vi "PAC-SLI.vi"() -> ()   [LabVIEW 2017]
uses:
  <vilib>/MakerHub/LINX/Private/Type Defs/Peripherals/SPI/SPI Configuration.ctl
  <vilib>/MakerHub/LINX/Private/Type Defs/Peripherals/SPI/SPI Bit Order.ctl
  <vilib>/MakerHub/LINX/Private/Type Defs/Peripherals/SPI/SPI Mode.ctl
  <vilib>/MakerHub/LINX/Public/Peripherals/SPI/SPI CS Config.ctl
  <vilib>/MakerHub/LINX/Private/Type Defs/Peripherals/SPI/SPI CS Logic Level.ctl
  <vilib>/Analysis/Matrix/Datatypes/RealMatrix.ctl
  <vilib>/MakerHub/LINX/Public/Peripherals/PWM/PWM Set Duty Cycle 1 Chan.vi
  <vilib>/MakerHub/LINX/Public/Peripherals/Analog/Analog Read 1 Chan.vi
  <vilib>/MakerHub/LINX/Public/Peripherals/Analog/Analog Read N Chans.vi
  <vilib>/MakerHub/LINX/Private/Local IO/LinxAnalogRead.vi
  <vilib>/MakerHub/LINX/Public/Utilities/Check Channel.vi
  <vilib>/MakerHub/LINX/Public/Utilities/Open Serial.vi
  <vilib>/MakerHub/LINX/Public/Peripherals/PWM/PWM Set Duty Cycle N Chans.vi
  <vilib>/MakerHub/LINX/Private/Utilties/Generate Error.vi
  <vilib>/Analysis/Matrix/Numeric/Conversions/Matrix To Array - RM.vi
  <vilib>/MakerHub/LINX/LMH-LINX.lvlib
  <vilib>/Analysis/Matrix/NI_Matrix.lvlib
panel:
  in  "START Button":bool
  out "stop 2":bool
  out "Connection Initialized":bool
  out "Debug console":string
  in  "reset":bool
  in  "stop":bool
  out "I/O Device Name":string
  in  "?":T1(tab)
  in  "StayON 6":bool
  in  "StayON 5":bool
  in  "StayON 4":bool
  in  "StayON 3":bool
  in  "StayON 2":bool
  in  "StayON 1":bool
  in  "Detector  6":bool
  out "Det 6 status":bool
  in  "Detector  5":bool
  out "Det 5 status":bool
  in  "Detector  4":bool
  out "Det 4 status":bool
  in  "Detector 3":bool
  out "Det 3 status":bool
  in  "Detector 2":bool
  out "Det 2 status":bool
  in  "Detector 1":bool
  out "Det 1 status":bool
  out "Photogate AIN":u8
  out "Stepper PUL DOUT":u8
  out "Stepper DIR DOUT":u8
  out "Stepper ENA DOUT":u8
  out "DigiPAC UART":u8
  out "Thermocouple 1":string
  out "Thermocouple 2":string
  out "Furnace ctrl Channel":u8
  out "Beam gate channel":u8
  in  "Furnace power% set":u8 max=100
  out "Furnace power%":u8
  out "Elapsed Super\nCycle Time (s)":dbl caption="Elapsed Time (s)"
  in  "Supercycle time [s]":dbl
  in  "CS Configuration":T2={"CS Channel"=7, "CS Logic Level"=enum."Active High"}
  in  "SPI Configuration":T4={"Clock Frequency"=1000000, "Bit Order"=enum."LSb First", "SPI Mode"=enum."Mode 0"}
  out "Clock Frequency":u32
  in  "CS Configuration 2":T2={"CS Channel"=7, "CS Logic Level"=enum."Active High"}
  in  "Photogate AIN":u8
  in  "Stepper PUL DOUT":u8
  in  "Stepper DIR DOUT":u8
  in  "Stepper ENA DOUT":u8
  in  "DigiPAC UART":u8
  in  "Furnace ctrl Channel":u8=9 min=9 max=10
  in  "Beam gate channel":u8
  in  "Operation|Time":T7
  in  "Serial Port":refnum<visa-resource-name>="COM3"
  # "Check settings before running!"
  # "I/O Channels"
  # "Temperature"
  # "Set      Status"
  # "Furnace power output"
  # "DIN.............."
  # "Digital input"
  # "DOUT.........."
  # "Digital output"
  # "AIN.............."
  # "Analog input"
  # "UART..........."
  # "Serial port"
  # "I/O ports"
  # "Thermocouple SPI settings"
  # "Automation order and timing"
  # "Thermocouple SPI settings required by MAX31855 amplifier:\nCS Logic level.............Active Low\nBit Order......................MSb First\nSPI Mode.....................Mode 0\nClock Frequency........<15000000\n                                      12500 is ok\nMISO/Data port...........50\nCLK port.......................52"
  # "Operation command numbers\n0, No action\n1, Detector acq. ON\n2, Detector acq. OFF\n3, Furnace power set\n4, Beam gate OFF\n5, Beam gate ON\n6, Furnace position IN\n7, Furnace position OUT\n8, Detector status check"
  # "Furnace control\nChannel forced\nto 9 or 10 due\nhardware setup\nin firmware.\nMore information in \ndocumentation"
  # "Author: Mikko Kivekäs\nVersion: 0.2.0\nDate: 07/2019\nLicense: GPLv3\n\nThis program is created for PAC-SLI measurement setup in ISOLDE, CERN. This program is created for research use and should not be used in commercial applications.\n\nThis program is designed to be operated with Arduino Mega2560 I/O-board.  Communication between Arduino and this LabVIEW program uses serial communication over USB. MakerHub LINX library is used. https://www.labviewmakerhub.com/doku.php?id=libraries:linx:start\n\n\nIn monitoring tab user can monitor input and output values. Monitoring tab has also the control of detector data acquisition control. \n\nSettings tab contains all essential settings for running the measurement automation. There user can control I/O-ports, SPI settings and automation operation order and timing. SPI is used to read temperature values from MAX31855KASA+ thermocouple amplifier-adc. SPI MISO and CLK ports are fixed due Arduino design and stated under SPI-settings.\n\n     I/O type.....................I/O-port\n     -MISO/DO/Data.......50\n     -CLK/Clock...............52\n\nFurnace power setting I/O-port must be digital I/O-port with PMW. Choose of digital ports 2-13 (Arduino Mega2560). \n\nIndicator next to device name is ON when link between PC and Arduino is established and ready to run. Spress Start-button to run.\n\nCAUTION! FURNACE MUST BE IN UP POSITION, OTHERWISE FURNACE WILL BREAK DURING RUN.\n\nIf program does not run normally or you press \"Abort Execution\" of LabVIEW, build firmware to Arduino again. It is good practice to build firmware before\nevery run start. One can build firmware in LabVIEW going \n\n    Tools >> MakerHUB >> LINX >> LINX Firmware Wizard...  \n\nand there choosing right I/O-board and communication channel. In case of firmware not installing properly, disconnect all wires from Arduino, go to Arduino \nIDE and build in empty Sketch. If that does uploads properly, you can proceed to build LINX firmware.\n\nYou can find VIs and other information from https://github.com/MikkoKivekas/PAC-SLI\n\nThis program uses custom LINX firmware, read more from README."
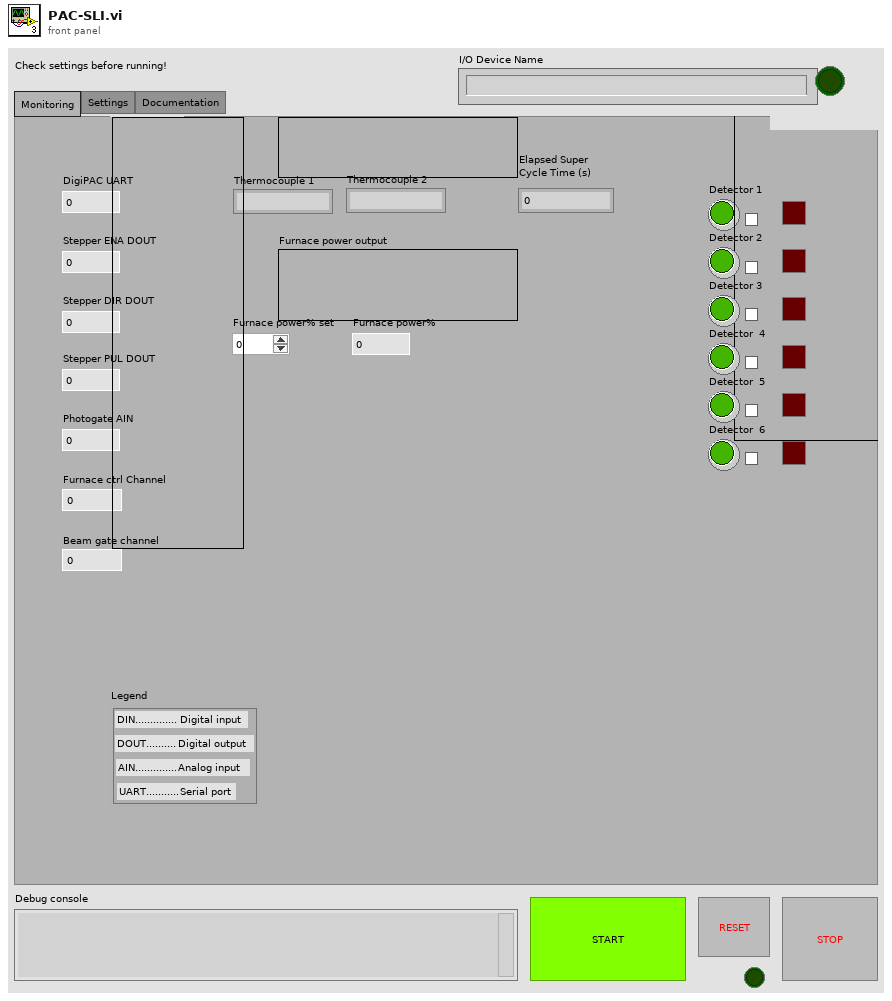
[diagram p1: front panel]
types:
  T1 = enum32{"Monitoring", "Settings", "Documentation"}
  T2 = typedef "LMH-LINX.lvlib/SPI CS Config.ctl" = cluster{"CS Channel":u8, "CS Logic Level":T3}
  T3 = typedef "LMH-LINX.lvlib/SPI CS Logic Level.ctl" = enum8{"Active Low", "Active High"}
  T4 = typedef "LMH-LINX.lvlib/SPI Configuration.ctl" = cluster{"Clock Frequency":u32, "Bit Order":T5, "SPI Mode":T6}
  T5 = typedef "LMH-LINX.lvlib/SPI Bit Order.ctl" = enum8{"LSb First", "MSb First"}
  T6 = typedef "LMH-LINX.lvlib/SPI Mode.ctl" = enum8{"Mode 0", "Mode 1", "Mode 2", "Mode 3"}
  T7 = typedef "NI_Matrix.lvlib/RealMatrix.ctl" = dbl[][]
  T8 = typedef "LMH-LINX.lvlib/LINX Ref.ctl" = cluster{"IO":T9, "Interface":T10, "LINX Device Config":T11}
  T9 = typedef "LMH-LINX.lvlib/Platform.ctl" = enum16{"Remote", "Local"}
  T10 = typedef "LMH-LINX.lvlib/Interface.ctl" = enum16{"Serial", "TCP"}
  T11 = typedef "LMH-LINX.lvlib/Device.lvlib/LINX Device Config.ctl" = cluster{"Interface":T10, "COM Port":refnum<visa-resource-name>, "TCP Configuration":T12, "Device Family":u8, "Device ID":u8, "Device Name":string, "TCP Ref":refnum<k5>, "Channels":T13}
  T12 = typedef "LMH-LINX.lvlib/Device.lvlib/TCP Config.ctl" = cluster{"IP Address":string, "Port":u16}
  T13 = typedef "LMH-LINX.lvlib/Channels.ctl" = cluster{"DI":u8[], "DO":u8[], "AI":u8[], "AO":u8[], "PWM":u8[], "QE":u8[], "UART":u8[], "I2C 2":u8[], "SPI":u8[], "CAN":u8[], "Servo":u8[], "AI Ref (V)":dbl, "AI Resolution (Bits)":u8, "AO Ref (V)":dbl, "AO Resolution (Bits)":u8}
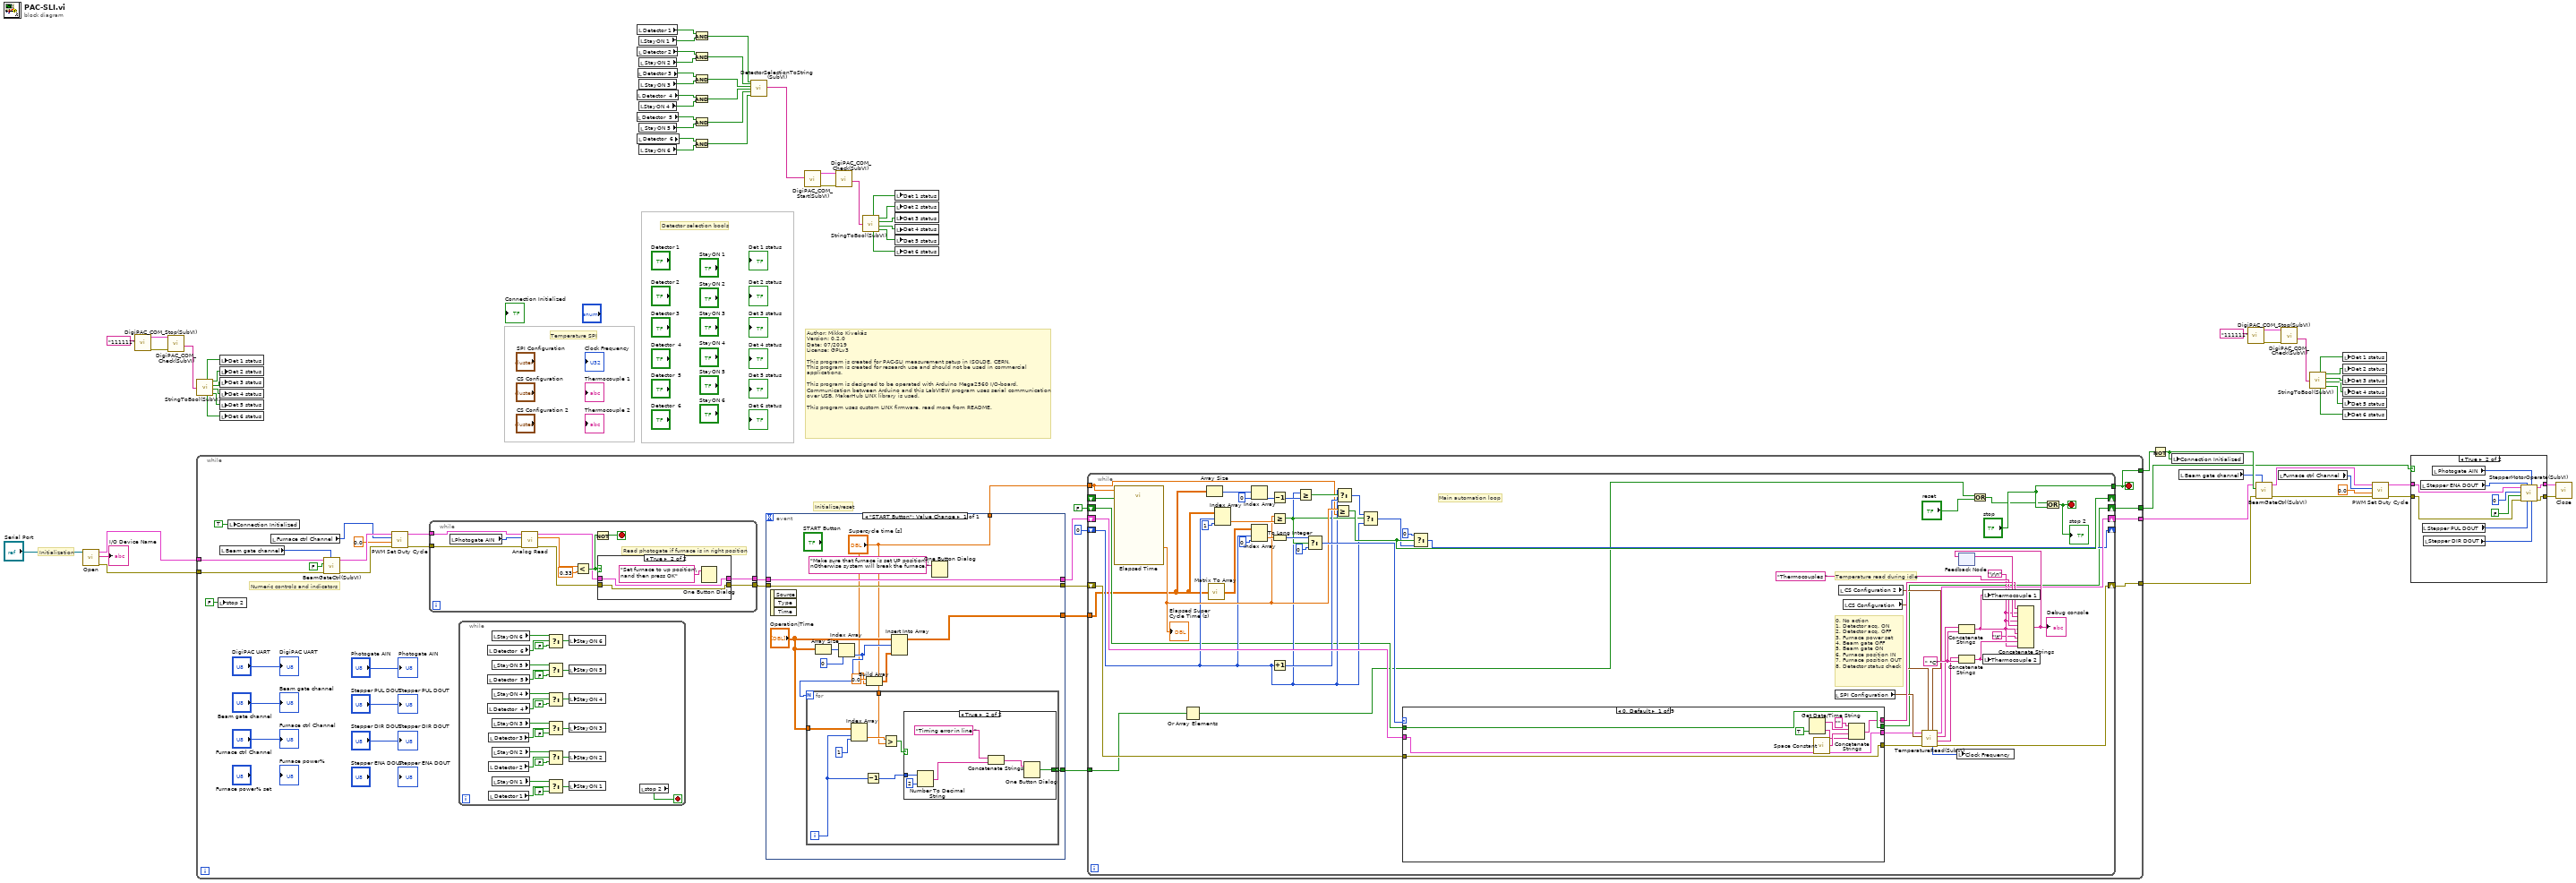
[diagram p0: block diagram]
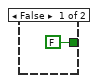
[diagram p4: hidden frame]
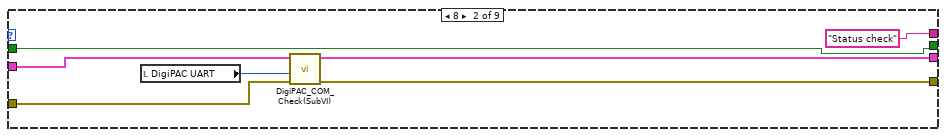
[diagram p5: hidden frame]
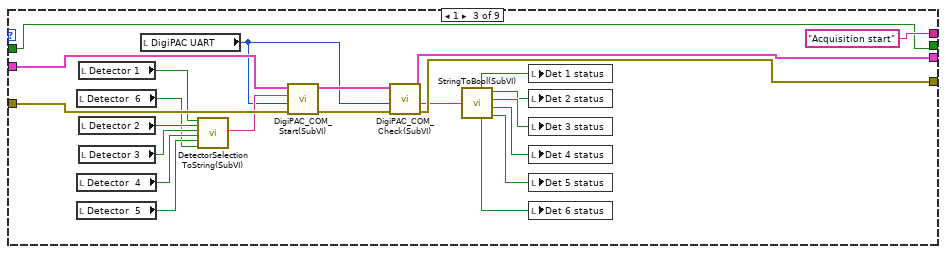
[diagram p6: hidden frame]
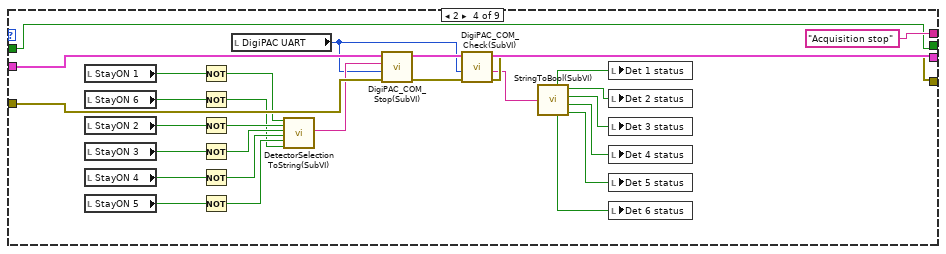
[diagram p7: hidden frame]
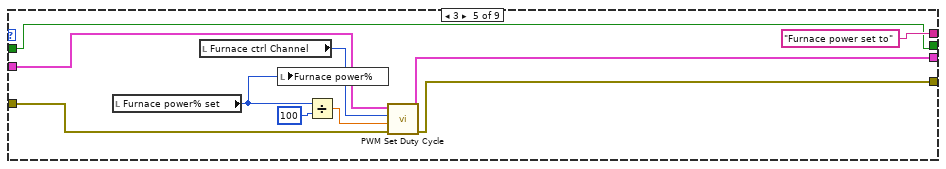
[diagram p8: hidden frame]
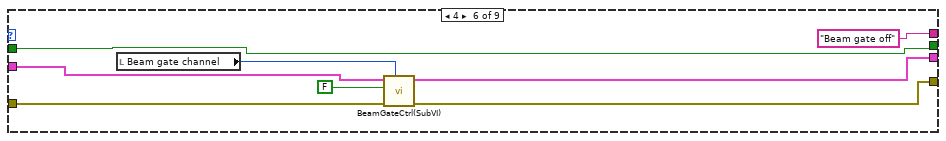
[diagram p9: hidden frame]
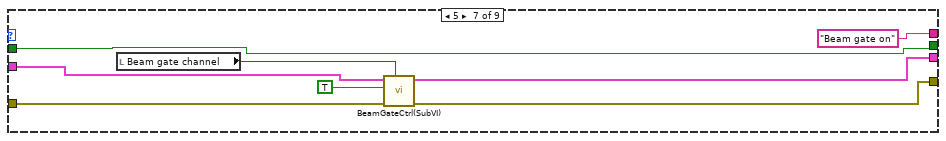
[diagram p10: hidden frame]
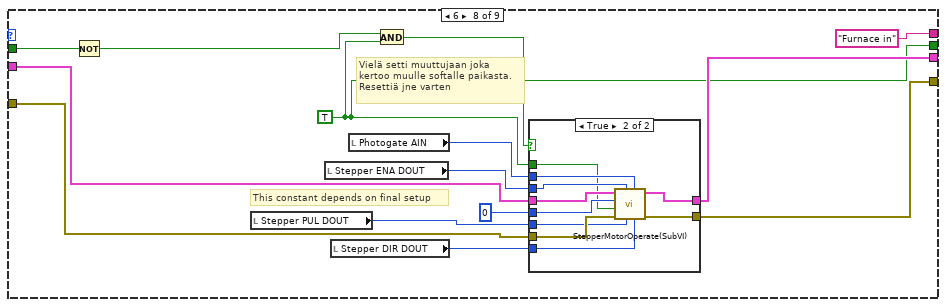
[diagram p11: hidden frame]
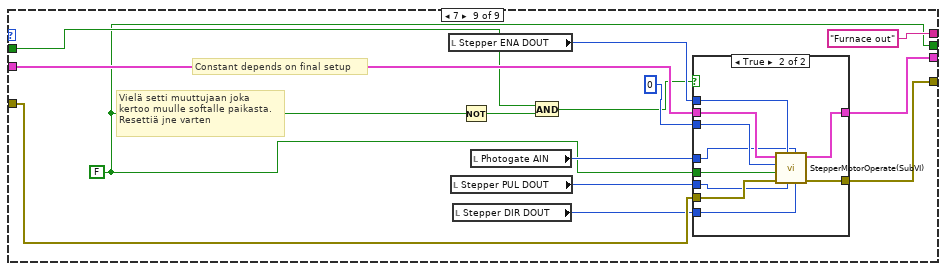
[diagram p13: hidden frame]
diagram:
  # "Author: Mikko Kivekäs\nVersion: 0.2.0\nDate: 07/2019\nLicense: GPLv3\n\nThis program is created for PAC-SLI measurement setup in ISOLDE, CERN.\nThis program is created for research use and should not be used in commercial\napplications.\n\nThis program is designed to be operated with Arduino Mega2560 I/O-board. \nCommunication between Arduino and this LabVIEW program uses serial communication\nover USB. MakerHub LINX library is used.\n\nThis program uses custom LINX firmware, read more from README."
  # "Initialization"
  # "Temperature SPI"
  # "Detector selection bools"
  n1 = call-poly <vilib>:"Open.vi"("Serial Port"="Serial Port") -> ("Error Out"=w63:errorcluster, "Device Name"=→"I/O Device Name":string, "LINX Resource"=w64:T8)  [unwired: 8 in]
  n2 = call "DigiPAC_COM_Stop(SubVI).vi"("Detector input"="111111") -> ("error out"=w37:errorcluster, "LINX Resource out"=w38:T8)  [unwired: 8 in, 1 out]
  n3 = call "DigiPAC_COM_Check(SubVI).vi"("error in (no error)"=w37, "LINX Resource in"=w38) -> ("Confirmation message"=w35:string)  [unwired: 6 in, 3 out]
  n4 = call "StringToBool(SubVI).vi"("string"=w35) -> ("Det 1"=w27:bool, "Det 2"=w26:bool, "Det 3"=w25:bool, "Det 6"=w22:bool, "Det 4"=w24:bool, "Det 5"=w23:bool)  [unwired: 4 in]
  n5 = while {
    tunnel: w64 -> [w83]
    tunnel: w63 -> [w82]
    tunnel: [w96] -> w59
    tunnel: [w95] -> w58
    tunnel: [w77] -> w62
    tunnel: [w91] -> w49
    stop <- w77 stop-if-true
    # "Numeric controls and indicators"
    # "Initialize/reset"
    n6 = local write "stop 2"(FALSE ("stop 2")) -> ()
    n7 = local read "Beam gate channel"() -> (w78:u8)
    n8 = local write "Connection Initialized"(TRUE ("Connection Initialized")) -> ()
    n9 = local read "Furnace ctrl Channel"() -> (w79:u8)
    n10 = call "BeamGateCtrl(SubVI).vi"("Beam gate ctrl channel"=w78, "Error In"=w82, "Output Value"=FALSE, "LINX Resource"=w83) -> ("Error Out"=w86:errorcluster, "LINX Resource 2"=w87:T8)  [unwired: 6 in]
    n11 = call-poly <vilib>:"PWM Set Duty Cycle.vi"("Error In"=w86, "Duty Cycle (0-1)"=0.0, "PWM Channel"=w79, "LINX Resource"=w87) -> ("Error Out"=w84:errorcluster, "LINX Resource"=w85:T8)  [unwired: 6 in]
    n12 = while {
      tunnel: w85 -> [w128]
      tunnel: [w126] -> w89
      tunnel: w84 -> [w125]
      tunnel: [w123] -> w88
      stop <- w129 stop-if-true
      # "Read photogate if furnace is in right position"
      n13 = local read "Photogate AIN"() -> (w131:u8)
      n14 = call-poly <vilib>:"Analog Read.vi"("Error In"=w125, "Analog Channel"=w131, "LINX Resource"=w128) -> ("Error Out"=w124:errorcluster, "Voltage"=w133:dbl, "LINX Resource"=w127:T8)  [unwired: 5 in, 1 out]
      n15 = Less?(x=w133, y=0.33) -> (x < y?=w130:bool)
      n16 = Not(x=w130) -> (.not. x?=w129:bool)
      n17 = case shown="True" w130 {
        tunnel: w127 -> [w135 w137]
        tunnel: [w135 w137] -> w126
        tunnel: w124 -> [w134 w136]
        tunnel: [w134 w136] -> w123
        frame False {
        }
        frame True {
          n18 = One Button Dialog(message="Set furnace to up position\nand then press OK") -> ()  [unwired: 1 in, 1 out]
        }
      }
    }
    n19 = while {
      stop <- w98 stop-if-true
      n20 = local read "Detector  6"() -> (w121:bool)
      n21 = local read "Detector  5"() -> (w119:bool)
      n22 = local read "Detector  4"() -> (w117:bool)
      n23 = local read "Detector 3"() -> (w115:bool)
      n24 = local read "Detector 2"() -> (w113:bool)
      n25 = local read "Detector 1"() -> (w111:bool)
      n26 = local read "StayON 6"() -> (w122:bool)
      n27 = local read "StayON 5"() -> (w120:bool)
      n28 = local read "StayON 4"() -> (w118:bool)
      n29 = local read "StayON 3"() -> (w116:bool)
      n30 = local read "StayON 2"() -> (w114:bool)
      n31 = local read "StayON 1"() -> (w112:bool)
      n32 = Select(t=w122, s=w121, f=FALSE) -> (s? t:f=w110:bool)
      n33 = Select(t=w120, s=w119, f=FALSE) -> (s? t:f=w109:bool)
      n34 = Select(t=w118, s=w117, f=FALSE) -> (s? t:f=w108:bool)
      n35 = Select(t=w116, s=w115, f=FALSE) -> (s? t:f=w107:bool)
      n36 = Select(t=w114, s=w113, f=FALSE) -> (s? t:f=w106:bool)
      n37 = Select(t=w112, s=w111, f=FALSE) -> (s? t:f=w105:bool)
      n38 = local write "StayON 6"(w110) -> ()
      n39 = local write "StayON 5"(w109) -> ()
      n40 = local write "StayON 4"(w108) -> ()
      n41 = local write "StayON 3"(w107) -> ()
      n42 = local write "StayON 2"(w106) -> ()
      n43 = local write "StayON 1"(w105) -> ()
      n44 = local read "stop 2"() -> (w98:bool)
    }
    n45 = event shown="[0] \"START Button\": Value Change" {
      selector: _ -> [_]
      dyn-events: _ -> [_]
      timeout: _ -> [_]
      tunnel: w89 -> [w149]
      tunnel: [w149] -> w94
      tunnel: w88 -> [w148]
      tunnel: [w148] -> w93
      tunnel: ["Supercycle time [s]"] -> w70
      tunnel: [w145] -> w68
      tunnel: [w139] -> w67
      event "START Button": Value Change {
        n46 = event-data() -> ()  [unwired: 1 in, 3 out]
        n47 = Array Size(array="Operation|Time") -> (size(s)=w144:i32[])
        n48 = Index Array(array=w144, index=0) -> (element=w142:i32)
        n49 = for {
          N: w142 -> [_]
          tunnel: "Operation|Time" -> [w158]
          tunnel: "Supercycle time [s]" -> [w155]
          tunnel: [w153] -> w139 mode=indexing
          i -> [w152]
          n50 = Index Array(array=w158, index (row)=w152, index (col)=1 ("disabled index (col)")) -> (element=w156:dbl)
          n51 = Decrement(x=w152) -> (x-1=w151:i32)
          n52 = Greater?(x=w156, y=w155) -> (0:w154:bool)
          n53 = case shown="True" w154 {
            tunnel: w151 -> [_ w165]
            tunnel: [FALSE ("true") w160] -> w153
            frame False {
            }
            frame True {
              n54 = Number To Decimal String(number=w165, width (-)=i16 2) -> (decimal integer string=w164:string)
              n55 = Concatenate Strings("Timing error in line ", w164) -> (w161:string)
              n56 = One Button Dialog(message=w161) -> (true=w160:bool)  [unwired: 1 in]
            }
          }
        }
        n57 = Build Array(0.0, "Supercycle time [s]") -> (w147:T7)
        n58 = Insert Into Array(array="Operation|Time", index (row)=w142, new element=w147) -> (w145:T7)  [unwired: 1 in]
        n59 = One Button Dialog(message="Make sure that furnace is set UP position.\nOtherwise system will break the furnace.") -> ()  [unwired: 1 in, 1 out]
      }
    }
    n60 = while {
      tunnel: ["stop"] -> w77
      shift-right: [w177] -> _
      shift-left: 0 -> [w176]
      shift-right: [w202] -> w96
      shift-left: w94 -> [w219]
      shift-right: [w201] -> w95
      shift-left: w93 -> [w218]
      shift-right: [w184] -> _
      shift-left: _ -> [w185]
      shift-right: [w175] -> w91
      shift-left: FALSE ("Direction input") -> [w174]
      tunnel: w70 -> [w173]
      tunnel: w68 -> [w171]
      tunnel: w67 -> [w170]
      stop <- w172 stop-if-true
      w188 = "\r\n"
      w213 = " °C"
      # "0, No action\n1, Detector acq. ON\n2, Detector acq. OFF\n3, Furnace power set\n4, Beam gate OFF\n5, Beam gate ON\n6, Furnace position IN\n7, Furnace position OUT\n8, Detector status check"
      # "Temperature read during idle"
      # "Main automation loop"
      n61 = call "Elapsed Time"("Time Target (s)"=w173, "Reset"=w185) -> ("Elapsed Time (s)"=w186:dbl)  [unwired: 10 in, 7 out]
      "Elapsed Super\nCycle Time (s)" <- w186
      n62 = Or Array Elements(Boolean array=w170) -> (logical OR=w168:bool)
      n63 = Array Size(array=w171) -> (size(s)=w217:i32[])
      n64 = call-poly <vilib>:"Matrix To Array.vi"("Real Matrix"=w171) -> ("Real 2D Array"=w215:dbl[][])
      n65 = Index Array(array=w171, index (row)=w176, index (col)=1 ("disabled index (col)")) -> (element=w195:dbl)
      n66 = Index Array(array=w217, index=0) -> (element=w210:i32)
      n67 = Index Array(array=w215, index (row)=w176, index (col)=0 ("disabled index (col)")) -> (element=w212:dbl)
      n68 = Decrement(x=w210) -> (x-1=w211:i32)
      n69 = Greater Or Equal?(x=w186, y=w195) -> (x >= y?=w179:bool)
      n70 = To Long Integer(number=w212) -> (32bit integer=w194:i32)
      n71 = Increment(x=w176) -> (x+1=w182:i32)
      n72 = Greater Or Equal?(x=w176, y=w211) -> (x >= y?=w181:bool)
      n73 = Select(t=w194, s=w179, f=0) -> (s? t:f=w192:i32)
      n74 = Greater Or Equal?(x=w186, y=w173) -> (x >= y?=w184:bool)
      n75 = Select(t=w176, s=w181, f=w182) -> (s? t:f=w180:i32)
      n76 = Select(t=w180, s=w179, f=w176) -> (s? t:f=w178:i32)
      n77 = case shown="0, Default" w192 {
        tunnel: w219 -> [w228 w234 w258 w287 w297 w305 w313 w327 w353]
        tunnel: [w228 w233 w256 w285 w296 w302 w310 w326 w352] -> w204
        tunnel: w218 -> [w227 w232 w255 w282 w295 w303 w311 w324 w350]
        tunnel: [w227 w231 w253 w284 w294 w301 w309 w325 w351] -> w203
        tunnel: [w223 "Status check" "Acquisition start" "Acquisition stop" "Furnace power set to" "Beam gate off" "Beam gate on" "Furnace in" "Furnace out"] -> w207
        tunnel: [w226 w229 w236 w259 w291 w298 w306 w315 w341] -> w175
        tunnel: w174 -> [w226 w229 w236 w259 w291 w298 w306 w316 w342]
        frame 0, Default {
          n78 = Get Date/Time String(want seconds? (F)=TRUE) -> (date string=w225:string, time string=w220:string)  [unwired: 2 in]
          n79 = call <vilib>:"Space Constant.vi"() -> ("String"=w221:string)
          n80 = Concatenate Strings("", w225, w221, w220) -> (w223:string)
        }
        frame 8 {
          n81 = local read "DigiPAC UART"() -> (w230:u8)
          n82 = call "DigiPAC_COM_Check(SubVI).vi"("error in (no error)"=w232, "UART Channel (0)"=w230, "LINX Resource in"=w234) -> ("error out"=w231:errorcluster, "LINX Resource out"=w233:T8)  [unwired: 5 in, 2 out]
        }
        frame 1 {
          n83 = local read "Detector  6"() -> (w239:bool)
          n84 = local read "Detector  4"() -> (w241:bool)
          n85 = local read "Detector  5"() -> (w240:bool)
          n86 = local read "Detector 1"() -> (w244:bool)
          n87 = local read "Detector 2"() -> (w243:bool)
          n88 = local read "Detector 3"() -> (w242:bool)
          n89 = local read "DigiPAC UART"() -> (w238:u8)
          n90 = call "DetectorSelectionToString(SubVI).vi"("Detector 1"=w244, "Detector 2"=w243, "Detector 3"=w242, "Detector 4"=w241, "Detector 5"=w240, "Detector 6"=w239) -> ("Output strting"=w245:string)  [unwired: 13 in]
          n91 = call "DigiPAC_COM_Start(SubVI).vi"("error in (no error)"=w255, "UART Channel (0)"=w238, "Detector input"=w245, "LINX Resource in"=w258) -> ("error out"=w254:errorcluster, "LINX Resource out"=w257:T8)  [unwired: 5 in, 1 out]
          n92 = call "DigiPAC_COM_Check(SubVI).vi"("error in (no error)"=w254, "UART Channel (0)"=w238, "LINX Resource in"=w257) -> ("error out"=w253:errorcluster, "Confirmation message"=w252:string, "LINX Resource out"=w256:T8)  [unwired: 5 in, 1 out]
          n93 = call "StringToBool(SubVI).vi"("string"=w252) -> ("Det 1"=w246:bool, "Det 2"=w247:bool, "Det 3"=w248:bool, "Det 6"=w251:bool, "Det 4"=w249:bool, "Det 5"=w250:bool)  [unwired: 4 in]
          n94 = local write "Det 1 status"(w246) -> ()
          n95 = local write "Det 2 status"(w247) -> ()
          n96 = local write "Det 3 status"(w248) -> ()
          n97 = local write "Det 4 status"(w249) -> ()
          n98 = local write "Det 5 status"(w250) -> ()
          n99 = local write "Det 6 status"(w251) -> ()
        }
        frame 2 {
          n100 = local read "StayON 1"() -> (w274:bool)
          n101 = local read "StayON 6"() -> (w269:bool)
          n102 = local read "StayON 2"() -> (w273:bool)
          n103 = local read "StayON 3"() -> (w272:bool)
          n104 = local read "StayON 4"() -> (w271:bool)
          n105 = local read "StayON 5"() -> (w270:bool)
          n106 = Not(x=w274) -> (.not. x?=w280:bool)
          n107 = Not(x=w269) -> (.not. x?=w275:bool)
          n108 = Not(x=w273) -> (.not. x?=w279:bool)
          n109 = Not(x=w272) -> (.not. x?=w278:bool)
          n110 = Not(x=w271) -> (.not. x?=w277:bool)
          n111 = Not(x=w270) -> (.not. x?=w276:bool)
          n112 = local read "DigiPAC UART"() -> (w267:u8)
          n113 = call "DetectorSelectionToString(SubVI).vi"("Detector 1"=w280, "Detector 2"=w279, "Detector 3"=w278, "Detector 4"=w277, "Detector 5"=w276, "Detector 6"=w275) -> ("Output strting"=w281:string)  [unwired: 13 in]
          n114 = call "DigiPAC_COM_Stop(SubVI).vi"("error in (no error)"=w282, "UART Channel (0)"=w267, "Detector input"=w281, "LINX Resource in"=w287) -> ("error out"=w283:errorcluster, "LINX Resource out"=w286:T8)  [unwired: 5 in, 1 out]
          n115 = call "DigiPAC_COM_Check(SubVI).vi"("error in (no error)"=w283, "UART Channel (0)"=w267, "LINX Resource in"=w286) -> ("error out"=w284:errorcluster, "Confirmation message"=w268:string, "LINX Resource out"=w285:T8)  [unwired: 5 in, 1 out]
          n116 = call "StringToBool(SubVI).vi"("string"=w268) -> ("Det 1"=w261:bool, "Det 2"=w262:bool, "Det 3"=w263:bool, "Det 6"=w266:bool, "Det 4"=w264:bool, "Det 5"=w265:bool)  [unwired: 4 in]
          n117 = local write "Det 1 status"(w261) -> ()
          n118 = local write "Det 2 status"(w262) -> ()
          n119 = local write "Det 3 status"(w263) -> ()
          n120 = local write "Det 4 status"(w264) -> ()
          n121 = local write "Det 5 status"(w265) -> ()
          n122 = local write "Det 6 status"(w266) -> ()
        }
        frame 3 {
          n123 = local read "Furnace power% set"() -> (w288:u8)
          n124 = local read "Furnace ctrl Channel"() -> (w293:u8)
          n125 = local write "Furnace power%"(w288) -> ()
          n126 = Divide(x=w288, y=u8 100) -> (x/y=w290:dbl)
          n127 = call-poly <vilib>:"PWM Set Duty Cycle.vi"("Error In"=w295, "Duty Cycle (0-1)"=w290, "PWM Channel"=w293, "LINX Resource"=w297) -> ("Error Out"=w294:errorcluster, "LINX Resource"=w296:T8)  [unwired: 6 in]
        }
        frame 4 {
          n128 = local read "Beam gate channel"() -> (w304:u8)
          n129 = call "BeamGateCtrl(SubVI).vi"("Beam gate ctrl channel"=w304, "Error In"=w303, "Output Value"=FALSE, "LINX Resource"=w305) -> ("Error Out"=w301:errorcluster, "LINX Resource 2"=w302:T8)  [unwired: 6 in]
        }
        frame 5 {
          n130 = local read "Beam gate channel"() -> (w312:u8)
          n131 = call "BeamGateCtrl(SubVI).vi"("Beam gate ctrl channel"=w312, "Error In"=w311, "Output Value"=TRUE, "LINX Resource"=w313) -> ("Error Out"=w309:errorcluster, "LINX Resource 2"=w310:T8)  [unwired: 6 in]
        }
        frame 6 {
          w315 = TRUE ("Direction input")
          # "Vielä setti muuttujaan joka \nkertoo muulle softalle paikasta.\nResettiä jne varten"
          # "This constant depends on final setup"
          n132 = Not(x=w316) -> (.not. x?=w317:bool)
          n133 = local read "Stepper PUL DOUT"() -> (w323:u8)
          n134 = local read "Stepper ENA DOUT"() -> (w320:u8)
          n135 = local read "Stepper DIR DOUT"() -> (w322:u8)
          n136 = local read "Photogate AIN"() -> (w319:u8)
          n137 = And(x=w317, y=w315) -> (x .and. y?=w314:bool)
          n138 = case shown="True" w314 {
            tunnel: w327 -> [w329 w339]
            tunnel: [w329 w338] -> w326
            tunnel: [w328 w337] -> w325
            tunnel: w324 -> [w328 w336]
            tunnel: w323 -> [_ w335]
            tunnel: w322 -> [_ w334]
            tunnel: 0 ("Maximum steps\ninput") -> [_ w333]
            tunnel: w320 -> [_ w332]
            tunnel: w319 -> [_ w331]
            tunnel: w315 -> [_ w330]
            frame False {
            }
            frame True {
              n139 = call "StepperMotorOperate(SubVI).vi"("DIR channel"=w334, "Photogate channel"=w331, "PUL channel"=w335, "ENA channel"=w332, "error in (no error)"=w336, "Direction input"=w330, "Maximum steps\ninput"=w333, "LINX Resource in"=w339) -> ("error out"=w337:errorcluster, "LINX Resource out"=w338:T8)  [unwired: 2 in]
            }
          }
        }
        frame 7 {
          w341 = FALSE ("Direction input")
          # "Vielä setti muuttujaan joka \nkertoo muulle softalle paikasta.\nResettiä jne varten"
          # "Constant depends on final setup"
          n140 = local read "Stepper ENA DOUT"() -> (w346:u8)
          n141 = local read "Stepper PUL DOUT"() -> (w349:u8)
          n142 = local read "Stepper DIR DOUT"() -> (w348:u8)
          n143 = Not(x=w341) -> (.not. x?=w343:bool)
          n144 = local read "Photogate AIN"() -> (w345:u8)
          n145 = And(x=w342, y=w343) -> (x .and. y?=w340:bool)
          n146 = case shown="True" w340 {
            tunnel: w353 -> [w355 w365]
            tunnel: [w355 w364] -> w352
            tunnel: [w354 w363] -> w351
            tunnel: w350 -> [w354 w362]
            tunnel: w349 -> [_ w361]
            tunnel: w348 -> [_ w360]
            tunnel: 0 ("Maximum steps\ninput") -> [_ w359]
            tunnel: w346 -> [_ w358]
            tunnel: w345 -> [_ w357]
            tunnel: w341 -> [_ w356]
            frame False {
            }
            frame True {
              n147 = call "StepperMotorOperate(SubVI).vi"("DIR channel"=w360, "Photogate channel"=w357, "PUL channel"=w361, "ENA channel"=w358, "error in (no error)"=w362, "Direction input"=w356, "Maximum steps\ninput"=w359, "LINX Resource in"=w365) -> ("error out"=w363:errorcluster, "LINX Resource out"=w364:T8)  [unwired: 2 in]
            }
          }
        }
      }
      n148 = Select(t=u8 0, s=w184, f=w178) -> (s? t:f=w177:i32)
      n149 = local read "SPI Configuration"() -> (w205:T4)
      n150 = local read "CS Configuration 2"() -> (w198:T2)
      n151 = local read "CS Configuration"() -> (w197:T2)
      n152 = call "TemperatureRead(SubVI).vi"("CS Configuration 2"=w198, "CS Configuration"=w197, "Error In"=w203, "SPI Configuration"=w205, "LINX Resource"=w204) -> ("Error Out"=w201:errorcluster, "Temp2"=w199:string, "Temp1"=w200:string, "LINX Resource 2"=w202:T8, "Actual Clock Frequency"=w206:u32)  [unwired: 2 in]
      n153 = local write "Clock Frequency"(w206) -> ()
      n154 = feedback #1() -> (w209:string)  [unwired: 1 in]
      n155 = Concatenate Strings(w200, w213) -> (w190:string)
      n156 = Concatenate Strings(w199, w213) -> (w189:string)
      n157 = Or(x=w168, y="reset") -> (x .or. y?=w166:bool)
      n158 = local write "Thermocouple 1"(w190) -> ()
      n159 = local write "Thermocouple 2"(w189) -> ()
      n160 = Concatenate Strings(w207, w188, w209, w188, "Thermocouples ", w188, w190, "\t", w189, w188) -> (w208:string)
      "Debug console" <- w208
      n161 = feedback-in #1(w208) -> ()
      n162 = Or(x=w166, y="stop") -> (x .or. y?=w172:bool)
      "stop 2" <- w172
    }
    "DigiPAC UART" <- "DigiPAC UART"
    "Furnace ctrl Channel" <- "Furnace ctrl Channel"
    "Beam gate channel" <- "Beam gate channel"
    "Stepper DIR DOUT" <- "Stepper DIR DOUT"
    "Stepper PUL DOUT" <- "Stepper PUL DOUT"
    "Photogate AIN" <- "Photogate AIN"
  }
  n163 = local write "Det 1 status"(w27) -> ()
  n164 = local write "Det 2 status"(w26) -> ()
  n165 = local write "Det 3 status"(w25) -> ()
  n166 = local write "Det 4 status"(w24) -> ()
  n167 = local write "Det 5 status"(w23) -> ()
  n168 = local write "Det 6 status"(w22) -> ()
  n169 = local read "Detector  4"() -> (w13:bool)
  n170 = local read "Detector  5"() -> (w11:bool)
  n171 = local read "Detector 1"() -> (w19:bool)
  n172 = local read "Detector 2"() -> (w17:bool)
  n173 = local read "Detector  6"() -> (w9:bool)
  n174 = local read "Detector 3"() -> (w15:bool)
  n175 = local read "StayON 1"() -> (w18:bool)
  n176 = local read "StayON 4"() -> (w12:bool)
  n177 = local read "StayON 2"() -> (w16:bool)
  n178 = local read "StayON 3"() -> (w14:bool)
  n179 = local read "StayON 5"() -> (w10:bool)
  n180 = local read "StayON 6"() -> (w8:bool)
  n181 = And(x=w19, y=w18) -> (x .and. y?=w7:bool)
  n182 = And(x=w17, y=w16) -> (x .and. y?=w6:bool)
  n183 = And(x=w15, y=w14) -> (x .and. y?=w5:bool)
  n184 = And(x=w13, y=w12) -> (x .and. y?=w4:bool)
  n185 = And(x=w11, y=w10) -> (x .and. y?=w3:bool)
  n186 = And(x=w9, y=w8) -> (x .and. y?=w2:bool)
  n187 = call "DetectorSelectionToString(SubVI).vi"("Detector 1"=w7, "Detector 2"=w6, "Detector 3"=w5, "Detector 4"=w4, "Detector 5"=w3, "Detector 6"=w2) -> ("Output strting"=w1:string)  [unwired: 13 in]
  n188 = call "DigiPAC_COM_Start(SubVI).vi"("Detector input"=w1) -> ("error out"=w20:errorcluster, "LINX Resource out"=w21:T8)  [unwired: 8 in, 1 out]
  n189 = call "DigiPAC_COM_Check(SubVI).vi"("error in (no error)"=w20, "LINX Resource in"=w21) -> ("Confirmation message"=w34:string)  [unwired: 6 in, 3 out]
  n190 = call "StringToBool(SubVI).vi"("string"=w34) -> ("Det 1"=w33:bool, "Det 2"=w32:bool, "Det 3"=w31:bool, "Det 6"=w28:bool, "Det 4"=w30:bool, "Det 5"=w29:bool)  [unwired: 4 in]
  n191 = local write "Det 1 status"(w33) -> ()
  n192 = local write "Det 2 status"(w32) -> ()
  n193 = local write "Det 3 status"(w31) -> ()
  n194 = local write "Det 4 status"(w30) -> ()
  n195 = local write "Det 5 status"(w29) -> ()
  n196 = local write "Det 6 status"(w28) -> ()
  n197 = Not(x=w62) -> (.not. x?=w61:bool)
  n198 = local write "Connection Initialized"(w61) -> ()
  n199 = local read "Beam gate channel"() -> (w55:u8)
  n200 = call "DigiPAC_COM_Stop(SubVI).vi"("Detector input"="111111") -> ("error out"=w52:errorcluster, "LINX Resource out"=w53:T8)  [unwired: 8 in, 1 out]
  n201 = call "BeamGateCtrl(SubVI).vi"("Beam gate ctrl channel"=w55, "Error In"=w58, "Output Value"=w61, "LINX Resource"=w59) -> ("Error Out"=w56:errorcluster, "LINX Resource 2"=w60:T8)  [unwired: 6 in]
  n202 = local read "Furnace ctrl Channel"() -> (w54:u8)
  n203 = call "DigiPAC_COM_Check(SubVI).vi"("error in (no error)"=w52, "LINX Resource in"=w53) -> ("Confirmation message"=w50:string)  [unwired: 6 in, 3 out]
  n204 = call "StringToBool(SubVI).vi"("string"=w50) -> ("Det 1"=w44:bool, "Det 2"=w43:bool, "Det 3"=w42:bool, "Det 6"=w39:bool, "Det 4"=w41:bool, "Det 5"=w40:bool)  [unwired: 4 in]
  n205 = local write "Det 1 status"(w44) -> ()
  n206 = local write "Det 2 status"(w43) -> ()
  n207 = local write "Det 3 status"(w42) -> ()
  n208 = local write "Det 4 status"(w41) -> ()
  n209 = local write "Det 5 status"(w40) -> ()
  n210 = local write "Det 6 status"(w39) -> ()
  n211 = call-poly <vilib>:"PWM Set Duty Cycle.vi"("Error In"=w56, "Duty Cycle (0-1)"=0.0, "PWM Channel"=w54, "LINX Resource"=w60) -> ("Error Out"=w47:errorcluster, "LINX Resource"=w48:T8)  [unwired: 6 in]
  n212 = case shown="True" w49 {
    tunnel: w48 -> [w367 w376]
    tunnel: w47 -> [w366 w377]
    tunnel: [w367 w375] -> w46
    tunnel: [w366 w374] -> w45
    frame False {
    }
    frame True {
      n213 = local read "Stepper ENA DOUT"() -> (w372:u8)
      n214 = local read "Stepper PUL DOUT"() -> (w369:u8)
      n215 = local read "Stepper DIR DOUT"() -> (w370:u8)
      n216 = local read "Photogate AIN"() -> (w371:u8)
      n217 = call "StepperMotorOperate(SubVI).vi"("DIR channel"=w370, "Photogate channel"=w371, "PUL channel"=w369, "ENA channel"=w372, "error in (no error)"=w377, "Direction input"=FALSE, "Maximum steps\ninput"=0 ("Maximum steps\ninput"), "LINX Resource in"=w376) -> ("error out"=w374:errorcluster, "LINX Resource out"=w375:T8)  [unwired: 2 in]
    }
  }
  n218 = call <vilib>:"Close.vi"("Error In"=w45, "LINX Resource"=w46) -> ()  [unwired: 9 in, 1 out]
